vi "Update_Model.vi"(8 "error in (no error)":errorcluster, 11 "IB_Settings_Item in":refnum<class "IB_Settings_Item.lvclass">) -> (0 "error out":errorcluster, 3 "IB_Settings_Item out":refnum<class "IB_Settings_Item.lvclass">)   [LabVIEW 2020, in "IB_Settings_Item.lvclass"]
uses:
  <vilib>/AppBuilder/IB_Classes/Settings_Item/IB_Settings_Item.lvclass
  <vilib>/AppBuilder/IB_Classes/Settings_Item/IB_Settings_Item.lvclass/IB_Settings_Item.ctl
  <vilib>/AppBuilder/IB_Classes/Installer/Installer.lvclass
  <vilib>/AppBuilder/IB_Classes/Source/Container/IB_Source_Container.lvclass
  <vilib>/AppBuilder/IB_Classes/Source/IB_Source.lvclass
  <vilib>/AppBuilder/IB_Classes/Destination/IB_Destination.lvclass
  <vilib>/AppBuilder/IB_Classes/Source/File/IB_Source_File.lvclass
  <vilib>/AppBuilder/IB_Classes/Source/File/CtrFile/IB_CtrFile.lvclass
  e:/builds/penguin/labview/branches/2020/dev/dist/vi.lib/AppBuilder/IB_Classes/Source/File/IB_Source_File.lvclass
  e:/builds/penguin/labview/branches/2020/dev/dist/vi.lib/AppBuilder/IB_Classes/Source/IB_Source.lvclass
  e:/builds/penguin/labview/branches/2020/dev/dist/vi.lib/AppBuilder/IB_Classes/Source/File/CtrFile/IB_CtrFile.lvclass
  e:/builds/penguin/labview/branches/2020/dev/dist/vi.lib/AppBuilder/IB_Classes/Source/Container/IB_Source_Container.lvclass
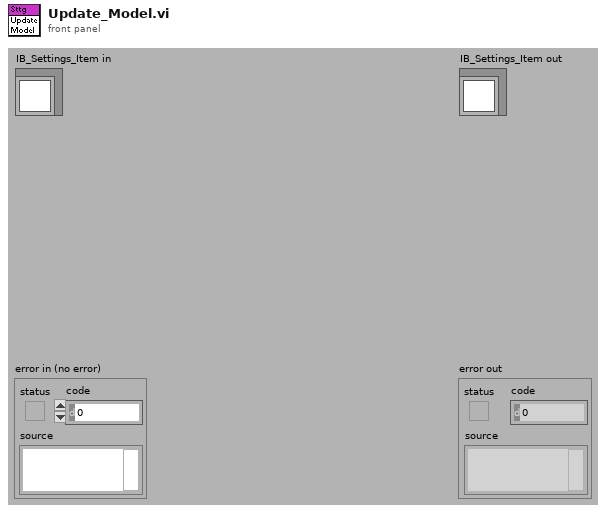
[diagram p1: front panel]
types:
  T1 = typedef "IB_Settings_Item.ctl" = cluster{"address":string[], "Attributes":i16, "RegCOM":bool, "unlock":bool}
  T2 = typedef "IB_Installer.ctl" = cluster{"Destination":refnum<class "IB_Destination.lvclass">[], "Source":refnum<class "IB_Source.lvclass">[], "buildObject":T3, "defaultDir":string, "platform":string, "author":string, "productName":string, "buildSpecName":string, "hide":bool, "requireLVDevSys":bool, "autoIncrement":bool, "includeError":bool, "readmeID":string, "buildLocation":path, "readmePath":path, "mediaSize":u16, "language":T4, "productVersion":T5, "preview":bool, "programmatic":bool, "progressBarEvents":T6, "userLog_Path":path, "shortcutAddresses":T8[], "EXE_Install Address":string, "EXE_Uninstall Address":string, "additional NIPaths":refnum<class "Dest_NI_NIPath.lvclass">[], "web service itemIDs":string[], "installerName":string}
  T3 = typedef "ItemRef.ctl" = u64
  T4 = typedef "CDK_sTypeDef_Languages.ctl" = u16
  T5 = typedef "CDK_sTypeDef_ProductVersion.ctl" = cluster{"Major":u8, "Minor":u8, "Update":u16}
  T6 = typedef "provcom_ProgressBar_Events.ctl" = cluster{"newJob":refnum<user-event>, "newItem":refnum<user-event>, "errorMsg":T7, "cancel":refnum<user-event>}
  T7 = typedef "mxLvBuildError.ctl" = refnum<user-event>
  T8 = typedef "CDK_sTypeDef_ShortcutAddress.ctl" = cluster{"file":string, "shortcut":string}
  T9 = typedef "IB_Destination.ctl" = cluster{"name":string, "unlock":bool, "parentTag":string, "destTag":string, "eng_installPath":string}
  T10 = typedef "IB_Source_File.ctl" = cluster{"Attributes":i16, "RegCOM":bool, "unlock":bool, "shortcuts":refnum<class "IB_Shortcut.lvclass">[], "EXE_install":bool, "CmdArg_install":string, "EXE_uninstall":bool, "CmdArg_uninstall":string}
  T11 = typedef "IB_Source_Container.ctl" = cluster{"files":refnum<class "IB_CtrFile.lvclass">[], "previewed?":bool, "preview error?":bool}
  T12 = typedef "IB_Source.ctl" = cluster{"name":string, "sourceTag":string, "destTag":string, "path":path, "eng_installPath":string, "UI_inBuild?":bool, "str ref?":bool}
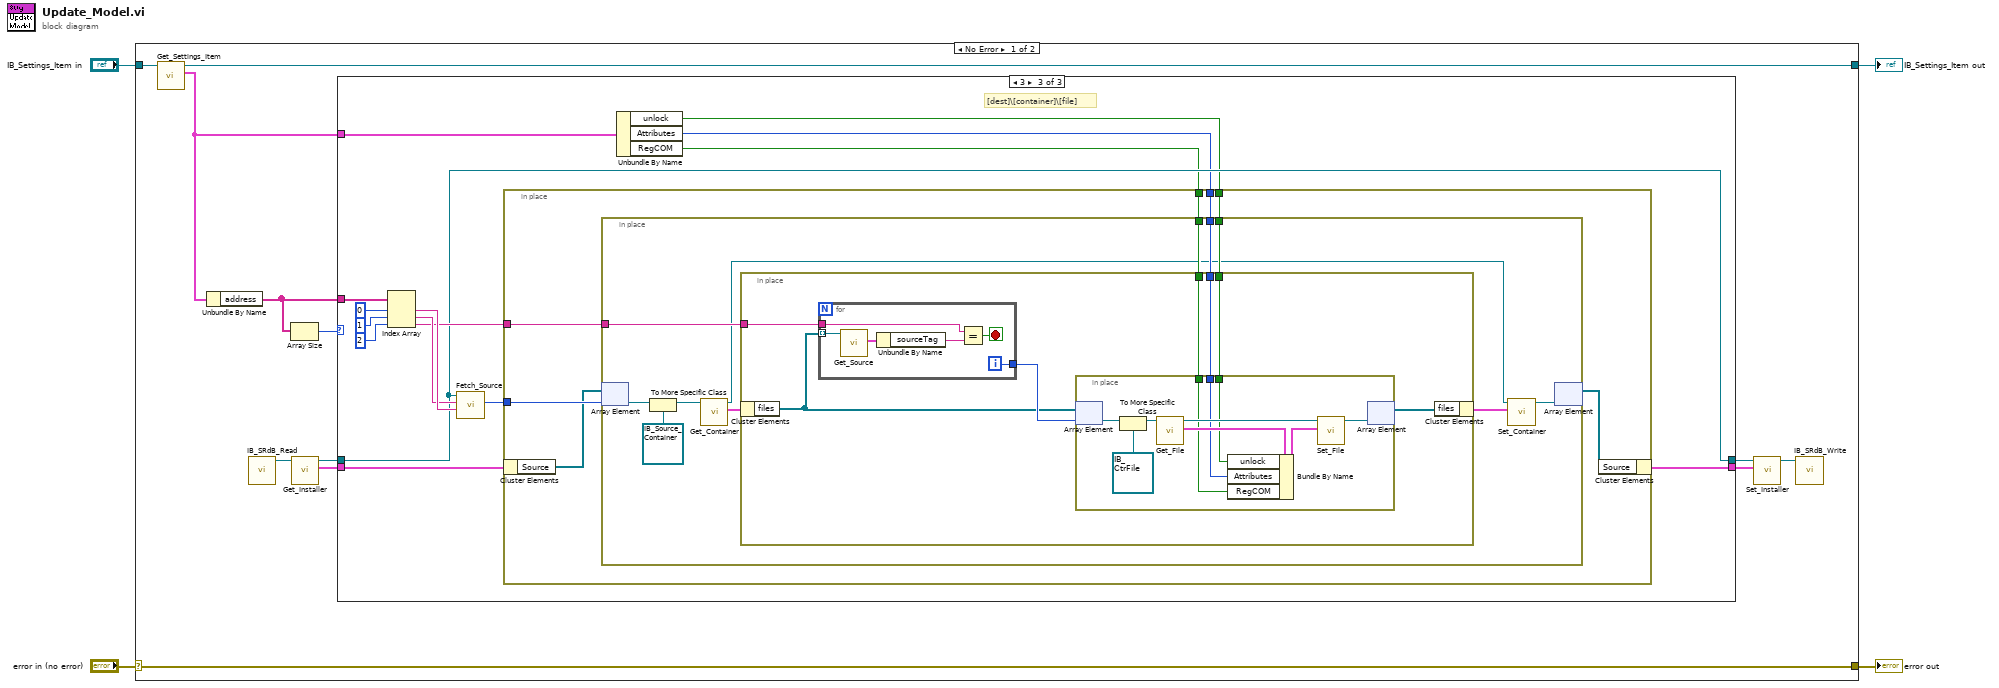
[diagram p0: block diagram]
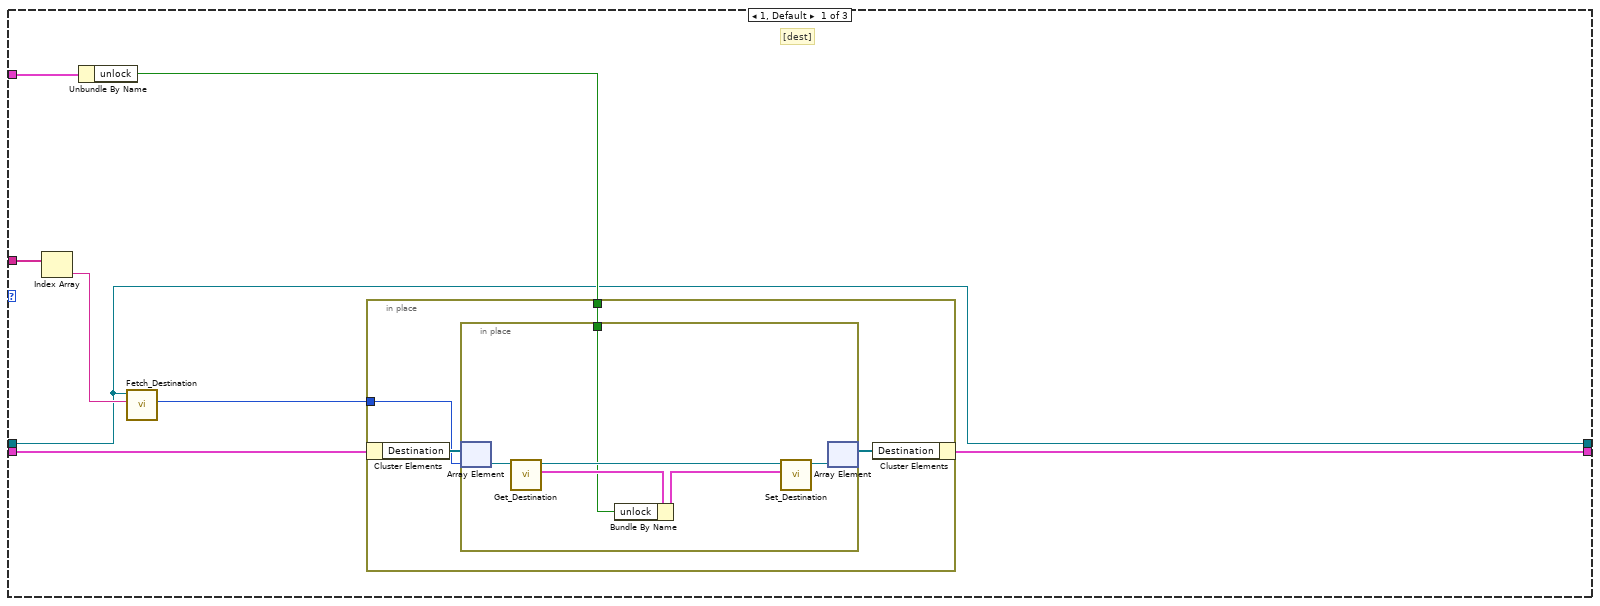
[diagram p2: hidden frame]
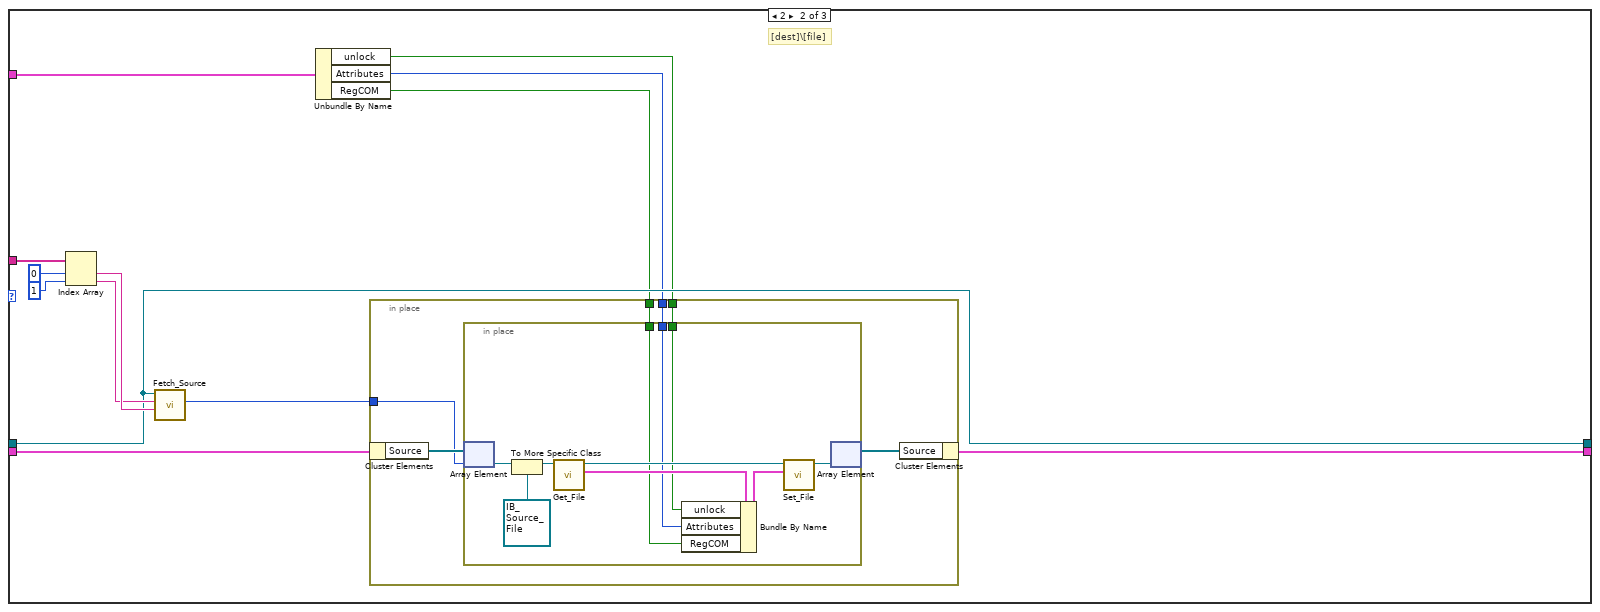
[diagram p3: hidden frame]
diagram:
  n1 = case shown="No Error" "error in (no error)" {
    selector: "error in (no error)" -> [w16 w121]
    tunnel: [w16 w121] -> w3
    tunnel: [w14 w120] -> w1
    tunnel: "IB_Settings_Item in" -> [w15 w120]
    frame No Error {
      n2 = call <vilib>:"Get_Settings_Item.vi"("IB_Settings_Item in"=w15) -> ("data"=w11:T1, "IB_Settings_Item out"=w14:refnum<class "IB_Settings_Item.lvclass">)  [unwired: 8 in, 1 out]
      n3 = Unbundle By Name(w11) -> ("address"=w12:string[])
      n4 = call <resource>:"IB_SRdB_Read.vi"() -> ("installer out"=w10:refnum<class "Installer.lvclass">)  [unwired: 10 in, 1 out]
      n5 = Array Size(array=w12) -> (size(s)=w13:i32)
      n6 = call <vilib>:"Get_Installer.vi"("Installer in"=w10) -> ("data"=w8:T2, "Installer out"=w9:refnum<class "Installer.lvclass">)  [unwired: 8 in, 1 out]
      n7 = case shown="3" w13 {
        tunnel: w12 -> [w23 w43 w72]
        tunnel: w11 -> [w22 w42 w70]
        tunnel: w9 -> [w18 w39 w71]
        tunnel: w8 -> [w19 w41 w65]
        tunnel: [w18 w39 w71] -> w6
        tunnel: [w17 w38 w64] -> w5
        frame 1, Default {
          # "[dest]"
          n8 = Index Array(array=w23) -> (element=w24:string)  [unwired: 1 in]
          n9 = Unbundle By Name(w22) -> ("unlock"=w20:bool)
          n10 = call <vilib>:"Fetch_Destination.vi"("destTag"=w24, "Installer in"=w18) -> ("index"=w21:i32)  [unwired: 7 in, 2 out]
          n11 = in-place {
            in-place-border: w21 -> [w26]
            in-place-border: w20 -> [w25]
            n12 = in-place-cluster #1(w19) -> ("Destination"=w28:refnum<class "IB_Destination.lvclass">[])
            n13 = in-place {
              in-place-border: w25 -> [w29]
              n14 = in-place-array #2(w28, w26) -> (w34:refnum<class "IB_Destination.lvclass">)
              n15 = call <vilib>:"Get_Destination.vi"("IB_Destination in"=w34) -> ("data"=w31:T9, "IB_Destination out"=w33:refnum<class "IB_Destination.lvclass">)  [unwired: 8 in, 1 out]
              n16 = Bundle By Name(cluster=w31, "unlock"=w29) -> (w30:T9)
              n17 = call <vilib>:"Set_Destination.vi"("data"=w30, "IB_Destination in"=w33) -> ("IB_Destination out"=w32:refnum<class "IB_Destination.lvclass">)  [unwired: 8 in, 1 out]
              n18 = in-place-array #2(w32) -> (w27:refnum<class "IB_Destination.lvclass">[])  [unwired: 1 out]
            }
            n19 = in-place-cluster #1("Destination"=w27) -> (w17:T2)
          }
        }
        frame 2 {
          # "[dest]\\[file]"
          n20 = Index Array(array=w43, index #1=0 ("index"), index #2=1 ("index")) -> (element #1=w45:string, element #2=w44:string)
          n21 = call <vilib>:"Fetch_Source.vi"("destTag"=w45, "sourceTag"=w44, "Installer in"=w39) -> ("index"=w40:i32)  [unwired: 6 in, 2 out]
          n22 = Unbundle By Name(w42) -> ("unlock"=w37:bool, "Attributes"=w36:i16, "RegCOM"=w35:bool)
          n23 = in-place {
            in-place-border: w40 -> [w51]
            in-place-border: w37 -> [w50]
            in-place-border: w36 -> [w49]
            in-place-border: w35 -> [w48]
            n24 = in-place-cluster #3(w41) -> ("Source"=w53:refnum<class "IB_Source.lvclass">[])
            n25 = in-place {
              in-place-border: w50 -> [w59]
              in-place-border: w49 -> [w55]
              in-place-border: w48 -> [w54]
              n26 = in-place-array #4(w53, w51) -> (w58:refnum<class "IB_Source.lvclass">)
              n27 = To More Specific Class(target class=refnum<class "IB_Source_File.lvclass"> refnum ("IB_Source_File in"), reference=w58) -> (specific class reference=w57:refnum<class "IB_Source_File.lvclass">)  [unwired: 1 in, 1 out]
              n28 = call <vilib>:"Get_File.vi"("IB_Source_File in"=w57) -> ("data"=w61:T10, "IB_Source_File out"=w63:refnum<class "IB_Source_File.lvclass">)  [unwired: 8 in, 1 out]
              n29 = Bundle By Name(cluster=w61, "unlock"=w59, "Attributes"=w55, "RegCOM"=w54) -> (w60:T10)
              n30 = call <vilib>:"Set_File.vi"("data"=w60, "IB_Source_File in"=w63) -> ("IB_Source_File out"=w62:refnum<class "IB_Source_File.lvclass">)  [unwired: 8 in, 1 out]
              n31 = in-place-array #4(w62) -> (w52:refnum<class "IB_Source.lvclass">[])  [unwired: 1 out]
            }
            n32 = in-place-cluster #3("Source"=w52) -> (w38:T2)
          }
        }
        frame 3 {
          # "[dest]\\[container]\\[file]"
          n33 = Index Array(array=w72, index #1=0 ("index"), index #2=1 ("index"), index #3=2 ("index")) -> (element #1=w76:string, element #2=w75:string, element #3=w73:string)
          n34 = call <vilib>:"Fetch_Source.vi"("destTag"=w76, "sourceTag"=w75, "Installer in"=w71) -> ("index"=w66:i32)  [unwired: 6 in, 2 out]
          n35 = Unbundle By Name(w70) -> ("unlock"=w69:bool, "Attributes"=w68:i16, "RegCOM"=w67:bool)
          n36 = in-place {
            in-place-border: w73 -> [w85]
            in-place-border: w69 -> [w84]
            in-place-border: w68 -> [w83]
            in-place-border: w67 -> [w82]
            in-place-border: w66 -> [w81]
            n37 = in-place-cluster #5(w65) -> ("Source"=w80:refnum<class "IB_Source.lvclass">[])
            n38 = in-place {
              in-place-border: w85 -> [w94]
              in-place-border: w84 -> [w93]
              in-place-border: w83 -> [w92]
              in-place-border: w82 -> [w91]
              n39 = in-place-array #6(w80, w81) -> (w87:refnum<class "IB_Source.lvclass">)
              n40 = To More Specific Class(target class=refnum<class "IB_Source_Container.lvclass"> refnum ("IB_Source_Container.lvclass"), reference=w87) -> (specific class reference=w95:refnum<class "IB_Source_Container.lvclass">)  [unwired: 1 in, 1 out]
              n41 = call <vilib>:"Get_Container.vi"("IB_Source_Container in"=w95) -> ("data"=w90:T11, "IB_Source_Container out"=w88:refnum<class "IB_Source_Container.lvclass">)  [unwired: 8 in, 1 out]
              n42 = in-place {
                in-place-border: w94 -> [w103]
                in-place-border: w93 -> [w101]
                in-place-border: w92 -> [w100]
                in-place-border: w91 -> [w99]
                n43 = in-place-cluster #7(w90) -> ("files"=w98:refnum<class "IB_CtrFile.lvclass">[])
                n44 = for {
                  tunnel: w103 -> [w116]
                  tunnel: w98 -> [w119] mode=indexing
                  tunnel: [w114] -> w102
                  i -> [w114]
                  stop <- w115 stop-if-true
                  n45 = call <vilib>:"Get_Source.vi"("IB_Source in"=w119) -> ("data"=w118:T12)  [unwired: 8 in, 2 out]
                  n46 = Unbundle By Name(w118) -> ("sourceTag"=w117:string)
                  n47 = Equal?(x=w116, y=w117) -> (x = y?=w115:bool)
                }
                n48 = in-place {
                  in-place-border: w101 -> [w110]
                  in-place-border: w100 -> [w107]
                  in-place-border: w99 -> [w106]
                  n49 = in-place-array #8(w98, w102) -> (w109:refnum<class "IB_CtrFile.lvclass">)
                  n50 = To More Specific Class(target class=refnum<class "IB_CtrFile.lvclass"> refnum ("IB_CtrFile.lvclass"), reference=w109) -> (specific class reference=w108:refnum<class "IB_CtrFile.lvclass">)  [unwired: 1 in, 1 out]
                  n51 = call <vilib>:"Get_File.vi"("IB_Source_File in"=w108) -> ("data"=w112:T10, "IB_Source_File out"=w113:refnum<class "IB_CtrFile.lvclass">)  [unwired: 8 in, 1 out]
                  n52 = Bundle By Name(cluster=w112, "unlock"=w110, "Attributes"=w107, "RegCOM"=w106) -> (w111:T10)
                  n53 = call <vilib>:"Set_File.vi"("data"=w111, "IB_Source_File in"=w113) -> ("IB_Source_File out"=w104:refnum<class "IB_CtrFile.lvclass">)  [unwired: 8 in, 1 out]
                  n54 = in-place-array #8(w104) -> (w97:refnum<class "IB_CtrFile.lvclass">[])  [unwired: 1 out]
                }
                n55 = in-place-cluster #7("files"=w97) -> (w89:T11)
              }
              n56 = call <vilib>:"Set_Container.vi"("data"=w89, "IB_Source_Container in"=w88) -> ("IB_Source_Container out"=w86:refnum<class "IB_Source_Container.lvclass">)  [unwired: 8 in, 1 out]
              n57 = in-place-array #6(w86) -> (w79:refnum<class "IB_Source.lvclass">[])  [unwired: 1 out]
            }
            n58 = in-place-cluster #5("Source"=w79) -> (w64:T2)
          }
        }
      }
      n59 = call <vilib>:"Set_Installer.vi"("data"=w5, "Installer in"=w6) -> ("Installer out"=w7:refnum<class "Installer.lvclass">)  [unwired: 8 in, 1 out]
      n60 = call <resource>:"IB_SRdB_Write.vi"("installer"=w7) -> ()  [unwired: 10 in, 1 out]
    }
    frame Error {
    }
  }
  "error out" <- w3
  "IB_Settings_Item out" <- w1
